vi "Read Settings path.vi"(8 "error in (no error)":errorcluster, 11 "Load-settings in":refnum<class "Load-settings.lvclass">) -> (0 "error out":errorcluster, 2 "Settings path":path, 3 "Load-settings out":refnum<class "Load-settings.lvclass">)   [LabVIEW 2013, in "SLMAPI.lvlib" / "Load-settings.lvclass"]
uses:
  Load-settings.lvclass
  Load-settings.lvclass/Load-settings.ctl
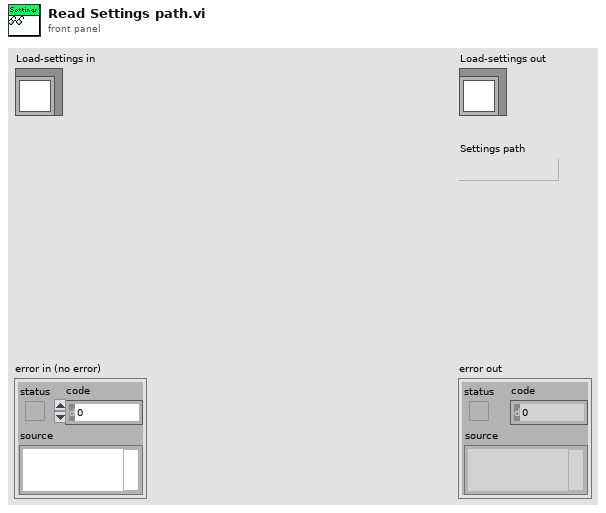
[diagram p1: front panel]
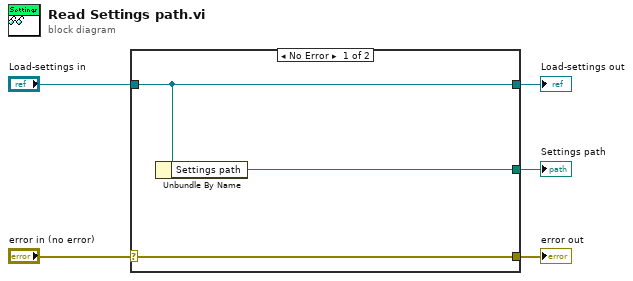
[diagram p0: block diagram]
diagram:
  n1 = case shown="No Error" "error in (no error)" {
    selector: "error in (no error)" -> [w8 w9]
    tunnel: [w8 w9] -> w4
    tunnel: [w7 w10] -> w2
    tunnel: "Load-settings in" -> [w7 w10]
    tunnel: [w6 _] -> w1
    frame No Error {
      n2 = Unbundle By Name(w7) -> ("Settings path"=w6:path)
    }
    frame Error {
    }
  }
  "error out" <- w4
  "Load-settings out" <- w2
  "Settings path" <- w1
